vi "GT Enable Do Bit Pulse.vi"(4 "firstLevel":i16, 5 "pulseNum":i32, 6 "lowLevelTime":u16, 7 "highLevelTime":u16, 8 "error in (no error)":errorcluster caption="错误输入（无错误）", 9 "doIndex":i16, 10 "doType":i16, 11 "cardNum":i16) -> (0 "error out":errorcluster caption="错误输出", 3 "function return":i16)   [LabVIEW 2014, in "gts.lvlib"]
doc: "GT_API GT_EnableDoBitPulse(short cardNum,short doType,short doIndex,unsigned short highLevelTime,unsigned short lowLevelTime,long pulseNum,short firstLevel);"
uses:
  gts.lvlib
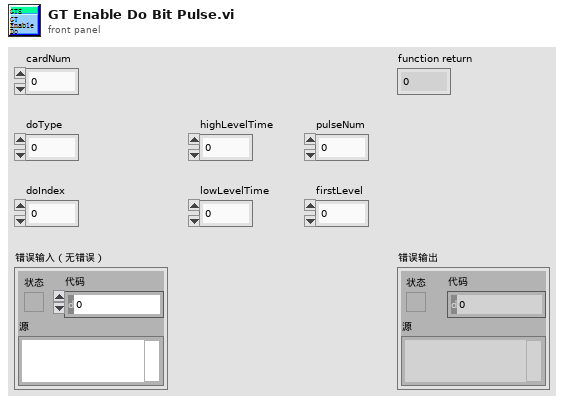
[diagram p1: front panel]
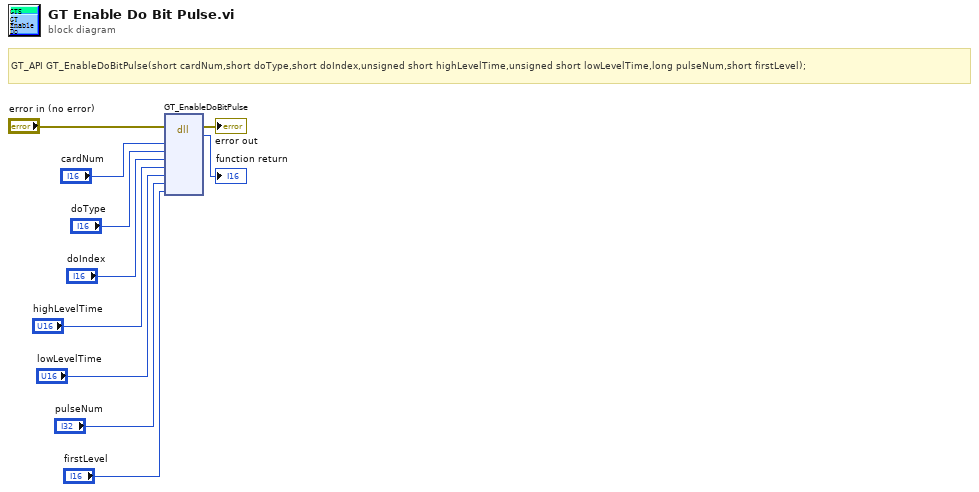
[diagram p0: block diagram]
diagram:
  # "GT_API GT_EnableDoBitPulse(short cardNum,short doType,short doIndex,unsigned short highLevelTime,unsigned short lowLevelTime,long pulseNum,short firstLevel);"
  n1 = dll-call lib="PTH2habs D固高科技资料GTS控制卡GTS卡18年上半年资料dllVC32bit\nmulti_cardgts.*" fn="GT_EnableDoBitPulse"(error in="error in (no error)", "cardNum"="cardNum", "doType"="doType", "doIndex"="doIndex", "highLevelTime"="highLevelTime", "lowLevelTime"="lowLevelTime", "pulseNum"="pulseNum", "firstLevel"="firstLevel") -> (error out=→"error out":errorcluster, →"function return":i16)  [unwired: 9 in, 1 out]
